vi "Run Test.vi"(8 "error in (no error)":errorcluster, 11 "Test Template in":refnum<class "LCM Single-Up Power Up.lvclass">) -> (0 "error out":errorcluster, 1 "Fail Codes":string[](array[string]), 2 "Tests Passed":bool[](array[boolean]), 3 "Test Template out":refnum<class "LCM Single-Up Power Up.lvclass">)   [LabVIEW 2015, in "LCM Single-Up Power Up.lvclass"]
uses:
  LCM Single-Up Power Up.lvclass
  Test Class/Test Class.lvclass/Test Class.ctl
  Test Class/Test Class.lvclass
  Classes/Application/Class/Application.lvclass
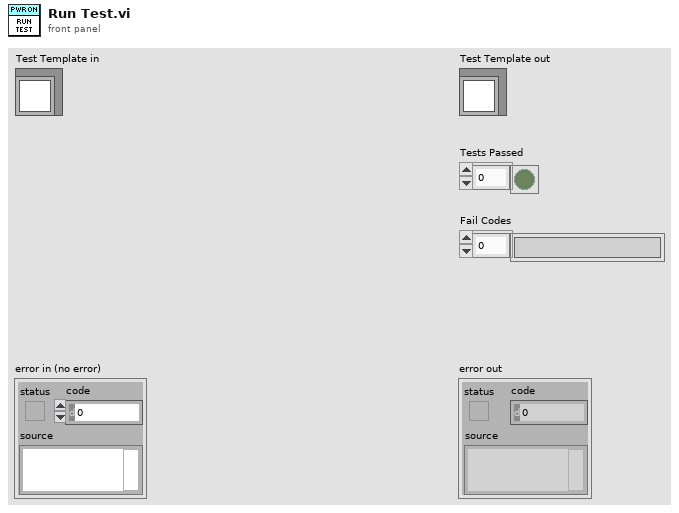
[diagram p1: front panel]
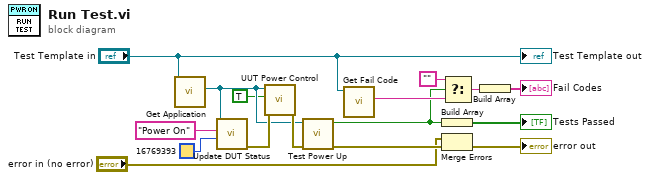
[diagram p0: block diagram]
diagram:
  n1 = call "Get Application.vi"("Test Class in"="Test Template in") -> ("Application.lvlib:Application.lvclass"=w2:refnum<class "Application.lvclass">)  [unwired: 9 in, 1 out]
  n2 = call "Update DUT Status.vi"("BG Color"=u32 16769393, "Message ('')"="Power On", "Application in"=w2) -> ("error out"=w3:errorcluster)  [unwired: 7 in, 1 out]
  n3 = call "UUT Power Control.vi"("error in (no error)"=w3, "Connect (False)"=TRUE, "Application in"=w2) -> ("error out"=w13:errorcluster)  [unwired: 8 in]
  n4 = call "Test Power Up.vi"("error in (no error)"=w13, "Application"=w2) -> ("error out"=w12:errorcluster, "result"=w7:bool)  [unwired: 8 in]
  n5 = call "Get Fail Code.vi"("Test Class in"="Test Template in") -> ("Fail Code"=w8:string)  [unwired: 9 in, 1 out]
  n6 = Build Array(w7) -> (→"Tests Passed":bool[])
  n7 = Merge Errors("error in (no error)", w12) -> (→"error out":errorcluster)
  n8 = Select(t="", s=w7, f=w8) -> (s? t:f=w5:string)
  n9 = Build Array(w5) -> (→"Fail Codes":string[])
  "Test Template out" <- "Test Template in"
